vi "Save.vi"(8 "error in":errorcluster, 10 "file path":path, 11 "repository in":refnum<class "CustomDeviceRepo.lvclass">) -> (0 "error out":errorcluster, 3 "repository out":refnum<class "CustomDeviceRepo.lvclass">)   [LabVIEW 2015, in "CustomDeviceRepo.lvclass"]
doc: "Stores repo information to file. It could save in multiple files or formats at the same time. File versioning is suggested."
uses:
  CustomDeviceRepo.lvclass
  NationalInstruments.VeriStand.XMLReader
  Configuration Tool.lvlib
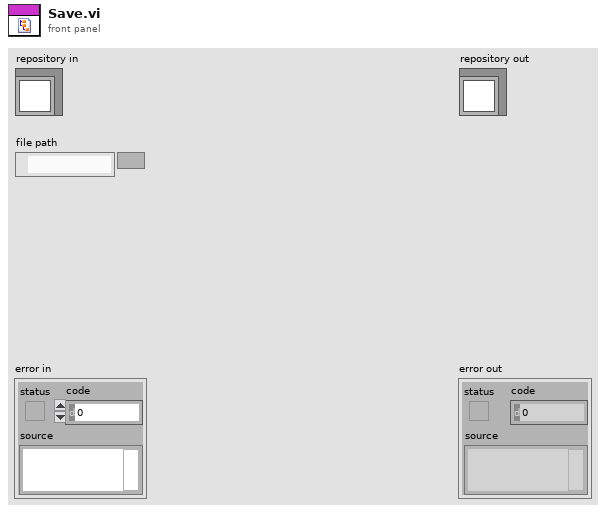
[diagram p1: front panel]
types:
  T1 = typedef "Main Custom Device Properties.ctl" = cluster{"CD Name":string, "Version":string, "Max Occurrences":i32, "Device Type":enum16{"Asynchronous", "Inline HW Interface", "Inline Model Interface", "Inline Timing and Sync", "Asynchronous Timing and Sync"}, "Main Page GUID":string}
  T2 = typedef "Initialization VI Properties.ctl" = cluster{"Execution":T3, "Path":T4, "Type":enum16{"Action", "VI"}, "Position":enum16{"centered", "mouse pointer"}}
  T3 = typedef "Configuration Tool.lvlib/Execution Types.ctl" = enum16{"silent", "modal", "floating", "default"}
  T4 = typedef "Configuration Tool.lvlib/Path Cluster.ctl" = cluster{"Path":path, "Path Type":enum16{"Absolute", "To Base", "To Common Doc Dir", "To Application Data Dir"}}
  T5 = typedef "Timing Source Properties.ctl" = cluster{"Has Timing Source Capability":bool, "Source Distribution":T6}
  T6 = typedef "Configuration Tool.lvlib/Source Distribution for TimingSource.ctl" = cluster{"Supported Target":T7, "Source":T4, "Real Time System Destination":string, "Version":string}[]
  T7 = typedef "Configuration Tool.lvlib/Target.ctl" = enum16{"All", "Pharlap", "VxWorks", "Windows", "Linux_32_ARM", "Linux_x64", "PharlapWindows", "PharlapVxWorks", "VxWorksWindows"}
  T8 = typedef "Configuration Tool.lvlib/Source Distribution for Custom Device VI.ctl" = cluster{"Source":T4, "Real Time System Destination":string, "Supported Target":T7}[]
  T9 = typedef "Page Properties.ctl" = cluster{"Name":string, "Disallow Renaming":bool, "Delete Protection":bool, "Exlcude from Alphabetical order":bool, "Allow Multi-Selection":bool, "GUID":string, "Parent GUIDs":string[], "Glyph":T4, "Inactive Glyph":T4, "Broken Glyph":T4, "Item to Launch":T4, "Additional Information":string, "Copy":enum16{"copy", "disabled"}, "Paste":enum16{"Create", "CreatIfNotExists_GUID", "CreatIfNotExists_Name", "Replace", "Dialog"}, "Help":T10}
  T10 = typedef "Configuration Tool.lvlib/help.ctl" = cluster{"Item to Launch":T4, "Section":string, "File Type":enum16{"chm", "other"}}
  T11 = typedef "ActionVIs Properties.ctl" = cluster{"Action VI On Delete":T4, "Action VI On Load":T4, "Action VI On Paste":T4, "Action VI On Target Type Change":T4, "Action VI On Delete Request":T4, "Action VI On Compile":T4, "Action VI On System Shutdown":T4, "Action VI On Save":T4, "Action VI On Download":T4}
  T12 = typedef "ButtonLists Properties.ctl" = cluster{"ID":string, "Glyph":T4, "Button Type":T13, "Referenced GUID":string, "Button Text":string, "Caption":string, "Tip Strip":string, "Documentation":string, "Dependency":T14}
  T13 = typedef "Configuration Tool.lvlib/Button Type.ctl" = enum16{"Action", "Dialog", "Page", "Notification", "Separator"}
  T14 = typedef "Configuration Tool.lvlib/Dependency three item small.ctl" = cluster{"File Path Control":path, "Path Type":enum16{"Absolute", "To Base", "To Common Doc Dir", "To Application Data Dir"}, "Behavior":enum16{"Static", "Dynamic"}}
  T15 = typedef "RunTimeMenus Properties.ctl" = cluster{"GUID":string, "Execution":T3, "MinNrOfChilds":u32, "Name":string, "Item to Launch":T4, "Dependency":T14, "Custom Population":T4, "Menu Item Type":enum16{"Action", "VI", "Separator", "Custom"}, "Behavior":enum16{"Nothing", "Open Front Panel"}, "Position":enum16{"Centered", "Mouse Pointer"}}
  T16 = cluster{"General Page Properties":T9, "ActionVIs Properties":T11, "Button List Properties":T12[], "RunTime Menus Properties":T15[]}[]
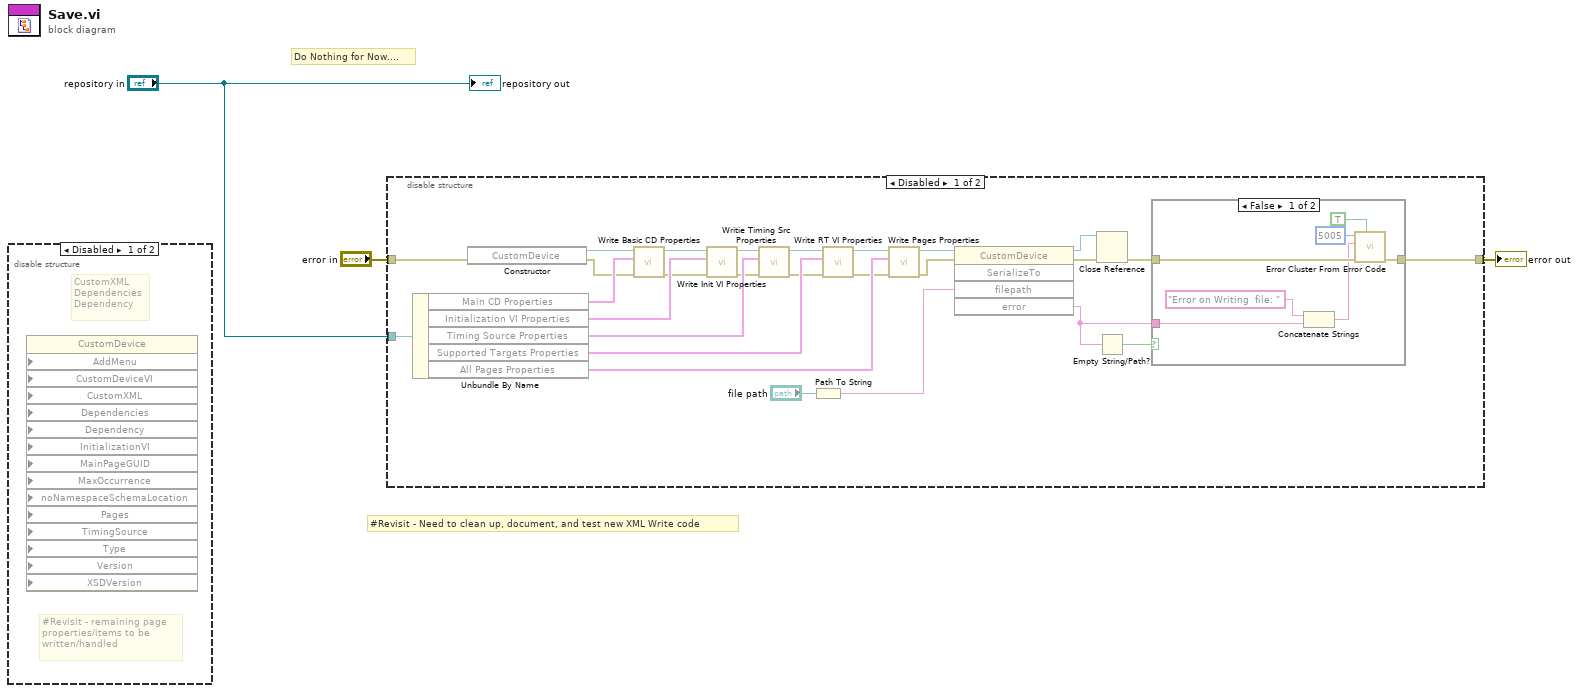
[diagram p0: block diagram]
diagram:
  # "#Revisit - Need to clean up, document, and test new XML Write code"
  # "Do Nothing for Now...."
  n1 = disable-structure shown="Disabled" {
    frame Disabled {
      # "#Revisit - remaining page\nproperties/items to be\nwritten/handled"
      # "CustomXML\nDependencies\nDependency"
      n2 = property class="CustomDevice" props=["AddMenu", "CustomDeviceVI", "CustomXML", "Dependencies", "Dependency", "InitializationVI", "MainPageGUID", "MaxOccurrence", "noNamespaceSchemaLocation", "Pages", "TimingSource", "Type", "Version", "XSDVersion"]() -> ()  [unwired: 16 in, 2 out]
    }
    frame Enabled {
    }
  }
  n3 = disable-structure shown="Disabled" {
    disable-tunnel: "repository in" -> [w30 _]
    disable-tunnel: "error in" -> [w14 w39]
    disable-tunnel: [w4 w39] -> w1
    frame Disabled {
      n4 = Unbundle By Name(w30) -> ("Main CD Properties"=w28:T1, "Initialization VI Properties"=w25:T2, "Timing Source Properties"=w22:T5, "Supported Targets Properties"=w19:T8, "All Pages Properties"=w16:T16)
      n5 = constructor class="CustomDevice"(error in=w14) -> (reference out=w29:refnum<k24>, error out=w27:errorcluster)  [unwired: 2 in, 1 out]
      n6 = call "Write Basic CD Properties.vi"("Error In"=w27, "Main CD Properties"=w28, "Custom Device .NET Ref In"=w29) -> ("Error Out"=w24:errorcluster, "Custom Device .NET Ref Out"=w26:refnum<k24>)  [unwired: 7 in]
      n7 = call "Write Init VI Properties.vi"("Error In"=w24, "Initialization VI Properties"=w25, "Custom Device .NET Ref In"=w26) -> ("Error Out"=w21:errorcluster, "Custom Device .NET Ref Out"=w23:refnum<k24>)  [unwired: 7 in]
      n8 = call "Writie Timing Src Properties.vi"("Error In"=w21, "Timing Source Properties"=w22, "Custom Device .NET Ref In"=w23) -> ("Error Out"=w18:errorcluster, "Custom Device .NET Ref Out"=w20:refnum<k24>)  [unwired: 7 in]
      n9 = Path To String(path="file path") -> (string=w11:string)
      n10 = call "Write RT VI Properties.vi"("Error In"=w18, "Supported Targets Properties"=w19, "Custom Device .NET Ref In"=w20) -> ("Error Out"=w15:errorcluster, "Custom Device .NET Ref Out"=w17:refnum<k24>)  [unwired: 7 in]
      n11 = call "Write Pages Properties.vi"("Error In"=w15, "All Pages Properties"=w16, "Custom Device .NET Ref In"=w17) -> ("Error Out"=w10:errorcluster, "Custom Device .NET Ref Out"=w13:refnum<k24>)  [unwired: 7 in]
      n12 = invoke class="CustomDevice" method="SerializeTo"(reference=w13, error in=w10, "filepath"=w11) -> (reference out=w7:refnum<k24>, error out=w6:errorcluster, "error"=w8:string)  [unwired: 2 in, 2 out]
      n13 = Close Reference(reference=w7, error in (no error)=w6) -> (error out=w5:errorcluster)
      n14 = Empty String/Path?(string/path=w8) -> (empty?=w9:bool)
      n15 = case shown="False" w9 {
        tunnel: w8 -> [w36 _]
        tunnel: w5 -> [w35 w38]
        tunnel: [w32 w38] -> w4
        frame False {
          n16 = Concatenate Strings("Error on Writing  file: " ("string"), w36) -> (w33:string)
          n17 = call <vilib>:"Error Cluster From Error Code.vi"("show call chain? (False)"=TRUE, "error in (no error)"=w35, "error message (\"\")"=w33, "error code (0)"=5005) -> ("error out"=w32:errorcluster)  [unwired: 5 in]
        }
        frame True {
        }
      }
    }
    frame Enabled {
    }
  }
  "error out" <- w1
  "repository out" <- "repository in"
